vi "Sub_Build_Connect_Flags_Byte.vi"(8 "error in (no error)":errorcluster, 11 "Connect Flags":T1) -> (0 "error out":errorcluster, 3 "ConnectFlags Byte":u8 format="%x")   [LabVIEW 2018, in "MQTT_Functions.lvlib"]
uses:
  MQTT_Functions.lvlib
  Controls/Connect_Flags.ctl
  Controls/QoS.ctl
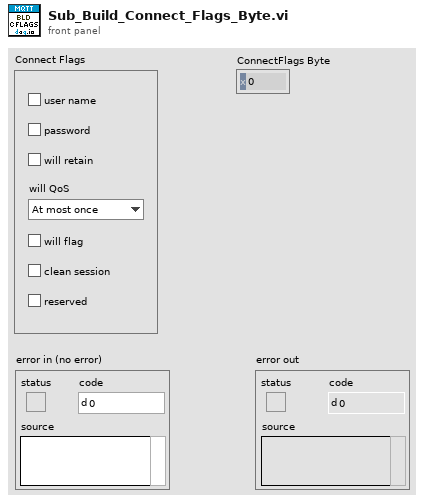
[diagram p1: front panel]
types:
  T1 = typedef "MQTT_Functions.lvlib/Connect_Flags.ctl" = cluster{"user name":bool, "password":bool, "will retain":bool, "will flag":bool, "clean session":bool, "reserved":bool, "will QoS":T2}
  T2 = typedef "MQTT_Functions.lvlib/QoS.ctl" = enum8{"At most once", "At least once", "Exactly once", "Reserved"}
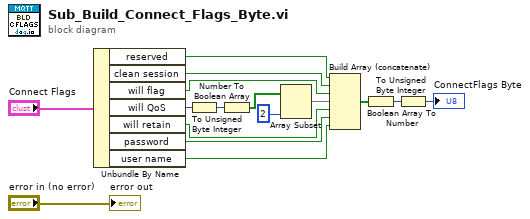
[diagram p0: block diagram]
diagram:
  n1 = Unbundle By Name("Connect Flags") -> ("reserved"=w12:bool, "clean session"=w11:bool, "will flag"=w10:bool, "will QoS"=w8:T2, "will retain"=w5:bool, "password"=w6:bool, "user name"=w7:bool)
  n2 = To Unsigned Byte Integer(number=w8) -> (unsigned 8bit integer=w16:u8)
  n3 = Number To Boolean Array(number=w16) -> (Boolean array=w15:bool[])
  n4 = Array Subset(array=w15, length=2) -> (w9:bool[])  [unwired: 1 in]
  n5 = Build Array (concatenate)(w12, w11, w10, w9, w5, w6, w7) -> (w4:bool[])
  n6 = Boolean Array To Number(Boolean array=w4) -> (number=w3:u32)
  n7 = To Unsigned Byte Integer(number=w3) -> (unsigned 8bit integer=→"ConnectFlags Byte":u8)
  "error out" <- "error in (no error)"
